vi "ReadMeasurements.vi"(5 "IP Address of SNMP Device":string, 6 "OID Numbers":string[](array[string]), 7 "Community Name":string, 8 "error in (no error)":errorcluster, 9 "Timeout(ms)":i32, 10 "Measurements To Read Array":u16[](array[numeric]), 11 "UDP Network Connection in":refnum<k16>) -> (0 "error out":errorcluster, 1 "SNMPDataAsStrings":string[][](array[string]), 3 "UDP Network Connection out":refnum<k16>)   [LabVIEW 2018, in "SensorPlugins.lvlib" / "RoomAlert.lvclass"]
doc: "Reads measurements from all the sensors."
uses:
  RoomAlert.lvclass
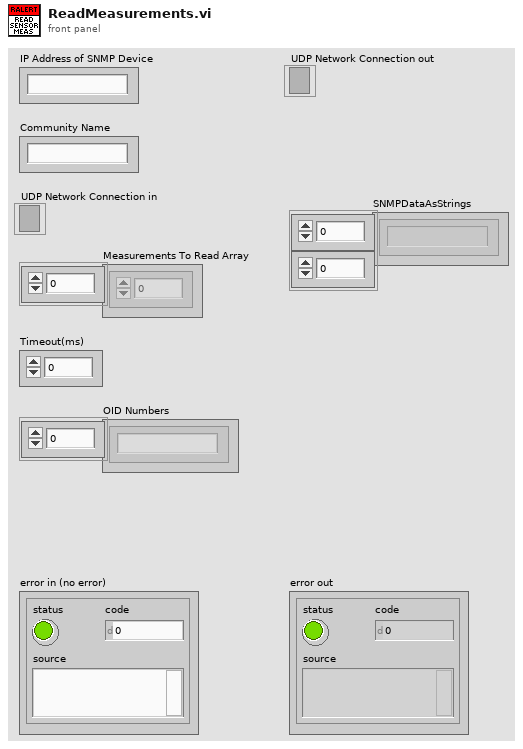
[diagram p1: front panel]
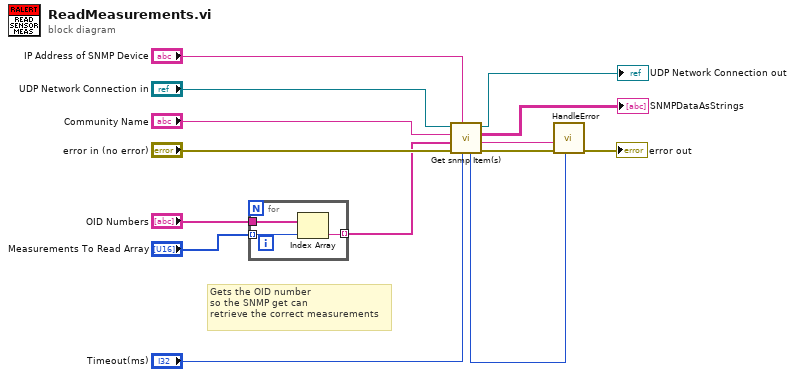
[diagram p0: block diagram]
diagram:
  # "Gets the OID number\nso the SNMP get can \nretrieve the correct measurements"
  n1 = for {
    tunnel: "Measurements To Read Array" -> [w16] mode=indexing
    tunnel: "OID Numbers" -> [w17]
    tunnel: [w15] -> w2 mode=indexing
    n2 = Index Array(array=w17, index=w16) -> (element=w15:string)
  }
  n3 = call "Get snmp Item(s).vi"("timeout ms (25000)"="Timeout(ms)", "IP Address of SNMP Device"="IP Address of SNMP Device", "error in (no error)"="error in (no error)", "OID ARRAY"=w2, "Community Name"="Community Name", "connection ID in"="UDP Network Connection in") -> ("error out"=w3:errorcluster, "error-string"=w6:string, "SnmpDataAsStrings"=→"SNMPDataAsStrings":string[][], "connection ID out"=→"UDP Network Connection out":refnum<k16>, "error-status"=w1:u8)  [unwired: 1 in]
  n4 = call "HandleError.vi"("error-status"=w1, "Error In"=w3, "Error String"=w6) -> ("Error Out"=→"error out":errorcluster)  [unwired: 8 in]
